vi "VectorTrigger6601.vi"(4 "pulse width (cycles)":i32=1, 5 "pulse polarity (high:0)":enum16{"high pulse ", "low pulse"}(ring), 6 "pulse delay (cycles)":i32=1, 8 "gate edge":T1(ring), 9 "source edge":T2(ring)) -> (1 "error out":errorcluster, 2 "task out":refnum<k21>)   [LabVIEW 2022 SP3]
doc: "Configures a counter to generate a single, delayed TTL pulse on its OUT pin. The signal is created by decrementing the counter twice, first for the delay to the pulse (called phase 1), then for the pulse itself (phase 2). The VI selects the highest resolution timebase for the counter to achieve the desired characteristics. You can optionally gate or trigger the operation with a signal on the counter's GATE pin. Call the Counter Start VI to start the pulse or enable it to be gated."
uses:
  <vilib>/DAQmx/create/channels.llb/DAQmx Create Channel (CO-Pulse Generation-Ticks).vi
  <vilib>/DAQmx/configure/trigger.llb/DAQmx Start Trigger (Digital Edge).vi
  <resource>/objmgr/daqmx.rc
panel:
  in  "error in (no error)":errorcluster
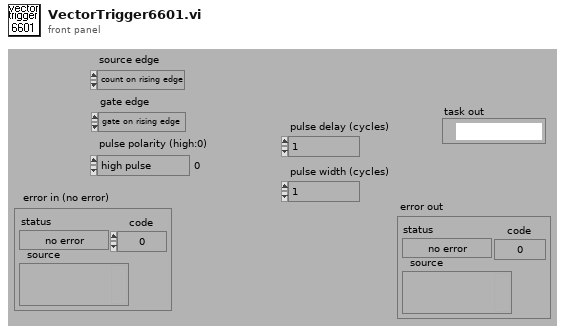
[diagram p1: front panel]
types:
  T1 = enum16{"gate on rising edge", "gate on falling edge"}
  T2 = enum16{"count on rising edge", "count on falling edge"}
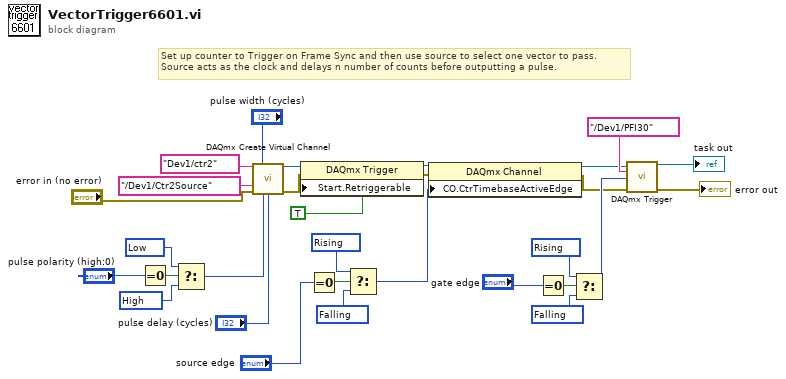
[diagram p0: block diagram]
diagram:
  w2 = 10214 items=["High"=10192, "Low"=10214] ("idle state")
  w1 = 10192 items=["High"=10192, "Low"=10214] ("idle state")
  w18 = 10171 items=["Rising"=10280, "Falling"=10171] ("edge")
  w19 = 10280 items=["Rising"=10280, "Falling"=10171] ("edge")
  w22 = 10171 items=["Rising"=10280, "Falling"=10171] ("ArmStart.DigEdge.Edge")
  w23 = 10280 items=["Rising"=10280, "Falling"=10171] ("ArmStart.DigEdge.Edge")
  # "Set up counter to Trigger on Frame Sync and then use source to select one vector to pass.\nSource acts as the clock and delays n number of counts before outputting a pulse."
  n1 = Equal To 0?(x="pulse polarity (high:0)") -> (x = 0?=w16:bool)
  n2 = Select(t=w2, s=w16, f=w1) -> (s? t:f=w15:i32)
  n3 = call-poly <vilib>:"DAQmx Create Virtual Channel.vi"("high ticks"="pulse width (cycles)", "counter"=tag "Dev1/ctr2", "source of ticks"=tag "/Dev1/Ctr2Source", "error in"="error in (no error)", "idle state"=w15, "initial delay"="pulse delay (cycles)") -> ("task out"=w8:refnum<k21>, "error out"=w7:errorcluster)  [unwired: 3 in, 5 out]
  n4 = property class="DAQmx Trigger"(reference=w8, error in=w7, "Start.Retriggerable"=TRUE) -> (reference out=w6:refnum<k21>, error out=w5:errorcluster)
  n5 = Equal To 0?(x="source edge") -> (x = 0?=w21:bool)
  n6 = Select(t=w23, s=w21, f=w22) -> (s? t:f=w10:i32)
  n7 = property class="DAQmx Channel"(reference=w6, error in=w5, "CO.CtrTimebaseActiveEdge"=w10) -> (reference out=w12:refnum<k21>, error out=w11:errorcluster)
  n8 = Equal To 0?(x="gate edge") -> (x = 0?=w20:bool)
  n9 = Select(t=w19, s=w20, f=w18) -> (s? t:f=w17:i32)
  n10 = call-poly <vilib>:"DAQmx Trigger.vi"("task/channels in"=w12, "source"=tag "/Dev1/PFI30", "edge"=w17, "error in"=w11) -> ("task out"=→"task out":refnum<k21>, "error out"=→"error out":errorcluster)  [unwired: 10 out]
